vi "BaseProvider_Configuration.vi"(1 "ClassRef/ClassPath(If empty Configuration default will be modified)":variant, 3 "OnlyWireStyleConfiguration(False)":bool, 5 "Error In":errorcluster) -> (15 "SelectedWireStyleIndex":i32, 19 "Error Out":errorcluster)   [LabVIEW 2020]
uses:
  Common/LvIcon_class/GDSLvIcon_ColorControl.ctl
  SubVIs/GOOP_WirePattern.ctl
  Common/ScriptingFunctions/Scripting_ConnectorPanePatternType.ctl
  BaseProvider_SubVIs/BaseProvider_WireStyleType.ctl
  SubVIs/GOOP_WireConfigurationType.ctl
  <vilib>/Utility/miscctls.llb/LVPositionTypeDef.ctl
  <vilib>/Utility/miscctls.llb/LVBoundsTypeDef.ctl
  Common/CommonVIs/CommonVIs_ClassIconSelection_Action.ctl
  BaseProvider_SubVIs/BaseProvider_FileNamingOption.ctl
panel:
  in  "File naming option":T1(ring)
  in  "WireStyleList":T2[](array[typedef])
  in  "DiscardChanges":bool
  in  "Update/AddWireStyle":bool
  in  "DeleteWireStyle":bool
  in  "Down":bool
  in  "Up":bool
  in  "WireStyleName":string caption="Selected Wire Style Name"
  out "ProductPicture":picture
  out "IconSelection":picture
  out "Icon":picture
  in  "_Dice":cluster{"Boolean 2":bool, "Dice 2":bool}
  in  "_DefaultConnectorPanePattern":T3 caption="Default Connector Pane Pattern" items=["4x4x4", "5x6x5", "6x8x6"]
  in  "_HelpDefaultConfiguration":bool
  in  "_Help":bool
  out "_ClassItemIconApperance":string caption="Class Item Icon Appearance"
  out "_WireApperance":string
  in  "_SetToDefaultForAllClasses":bool caption="Set this to default\nfor all future classes"
  in  "_Cancel":bool
  out "_Preview":picture caption="Preview"
  in  "_Icon":u16(ring) caption="Icon" items=["BlueFull", "BlueFrame", "InterfaceBlue", "BlueCircle", "BrownFull", "BrownFrame", "InterfaceBrown", "BrownCircle", "BurgundyFull", "BurgundyFrame", "InterfaceBurgundy", "BurgundyCircle", "CyanFull", "CyanFrame", "InterfaceCyan", "CyanCircle", "DarkBlueFull", "DarkBlueFrame", "InterfaceDarkBlue", "DarkBlueCircle", "ForestGreenFull", "ForestGreenFrame", "InterfaceForestGreen", "ForestGreenCircle", "GrayFull", "GrayFrame", "InterfaceGray", "GrayCircle", "GreenFull", "GreenFrame", "InterfaceGreen", "GreenCircle", "LightGreenFull", "LightGreenFrame", "InterfaceLightGreen", "LightGreenCircle", "LightRedFull", "LightRedFrame", "InterfaceLightRed", "LightRedCircle", "PinkFull", "PinkFrame", "InterfacePink", "PinkCircle", "PurpleFull", "PurpleFrame", "InterfacePurple", "PurpleCircle", "RedFull", "RedFrame", "InterfaceRed", "RedCircle", "YellowFull", "YellowFrame", "InterfaceYellow", "YellowCircle"]
  in  "_TunnelsAndTerminalsColors":T4 caption="Tunnels and \nTerminals Colors"
  in  "_CenterColor2":T4 caption="Pattern Colors"
  in  "_CenterColor1":T4 caption="Pattern Colors"
  in  "_CenterPattern":T5 caption="Center pattern"
  in  "_EdgeColor":T4 caption="Edge color"
  in  "_CenterThickness":T6(ring) caption="Center thickness"
  in  "_EdgeThickness":T7(ring) caption="Edge thickness"
  out "Wire preview":picture
  in  "_Done":bool
  # "Wire Configuration"
  # "Wire Appearance"
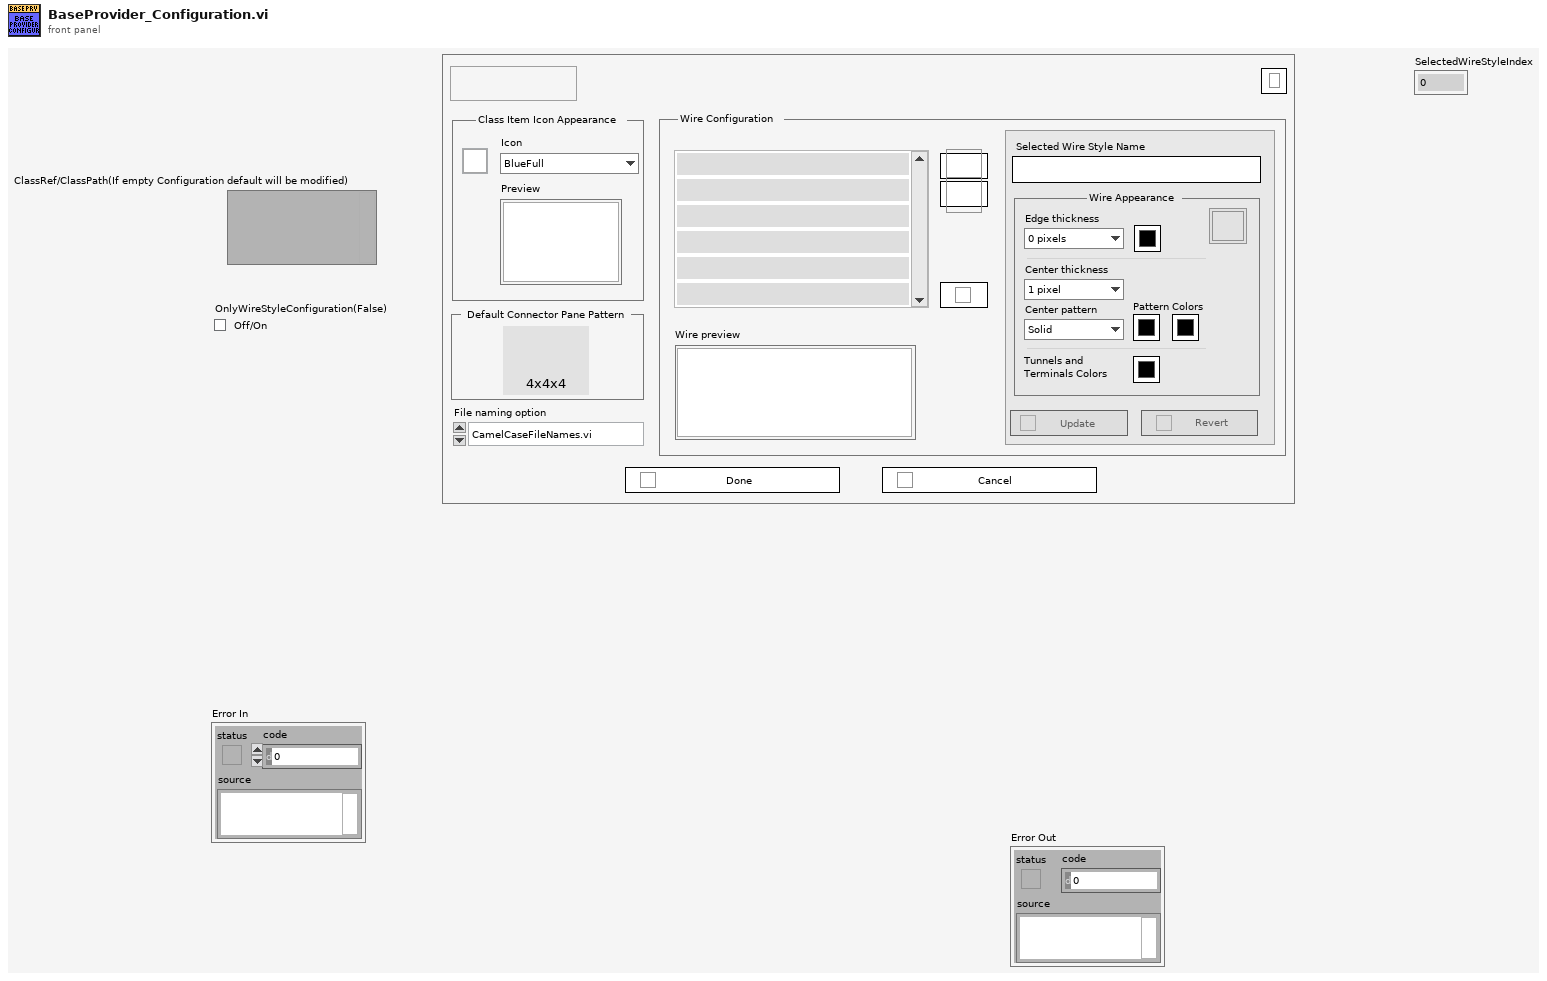
[diagram p1: front panel]
types:
  T1 = enum16{"CamelCaseFileNames.vi", "File Names With Spaces.vi", "File_Names_With_Underscores"}
  T2 = typedef "BaseProvider_WireStyleType.ctl" = cluster{"Boolean":bool, "Wire":picture, "Name":string, "Status":u16}
  T3 = typedef "Scripting_ConnectorPanePatternType.ctl" = u16
  T4 = typedef "GDSLvIcon_ColorControl.ctl" = cluster{"Decal":bool, "Color":u32}
  T5 = typedef "GOOP_WirePattern.ctl" = enum16{"Solid", "Large dash", "Small dash"}
  T6 = enum16{"1 pixel", "2 pixels", "3 pixels", "4 pixels", "5 pixels"}
  T7 = enum16{"0 pixels", "1 pixel", "2 pixels", "3 pixels"}
  T8 = typedef "GOOP_WireConfigurationType.ctl" = cluster{"Edge thickness":i32, "Edge color":u32, "Center thickness":i32, "Center pattern":T5, "CenterColor1":u32, "CenterColor2":u32, "Tunnels and terminals colors":u32}
  T9 = cluster{"FirstTime":bool, "ClassRef":refnum<vi>, "ClassRefCreated":bool, "CurrentWireStyle":T8, "DefaultIndex":i32, "SelectedWireStyleIndex":i32, "StartWireStyleIndex":i32}
  T10 = typedef "LVPositionTypeDef.ctl" = cluster{"Left":i32, "Top":i32}
  T11 = typedef "LVBoundsTypeDef.ctl" = cluster{"Width":u32, "Height":u32}
  T12 = typedef "BaseProvider_FileNamingOption.ctl" = enum16{"CamelCase", "Space", "Underscore"}
  T13 = typedef "BaseProvider_IniFileSettings.ctl" = cluster{"ClassFolderSuffix":string, "InterfaceFolderSuffix":string, "InterfaceIcon":string, "FileNamingOption":T12, "DynamicDispatchStartValue":bool, "UseGetSetForPropertyNodeMethods":bool}
  T14 = typedef "GDSLvCLass_ClassSettingsType.ctl" = cluster{"ClassProviderName":string, "ClassTemplateUsed":string, "ClassTemplateVersion":string, "ClassDescription":string, "PlugIns":T15[], "ConnectorPanePattern":string}
  T15 = typedef "GDSLvClass_PlugIn.ctl" = cluster{"Type":T16, "ID":string, "Version":string, "Path":path, "Name":string, "Data":variant}
  T16 = typedef "GDSLvClass_PlugInTypes.ctl" = enum16{"DesignPattern", "MethodTypes"}
  T17 = cluster{"Foreground Color":u32, "Background Color":u32, "Fill Pattern":cluster{"Row 0":u8, "Row 1":u8, "Row 2":u8, "Row 3":u8, "Row 4":u8, "Row 5":u8, "Row 6":u8, "Row 7":u8}, "Width":i16, "Mode":enum16{"Copy", "Or", "Exclusive Or", "Bit Clear", "Not Copy", "Not Or", "Nor Exclusive Or", "Not Bit Clear"}, "Style":enum32{"Solid", "Dash", "Dot", "Dash Dot", "Dash Dot Dot"}, "Fill Rule":enum32{"Even Odd", "Winding"}, "End Caps":enum32{"Default", "Flat"}}[]
  T18 = enum8{"Enabled", "Disabled", "Disabled and Grayed Out"}
  T19 = typedef "imagedata.ctl" = cluster{"image type":i32, "image depth":i32, "image":u8[], "mask":u8[], "colors":u32[], "Rectangle":cluster{"left":i16, "top":i16, "right":i16, "bottom":i16}}
  T20 = typedef "CommonVIs_ClassIconSelection_Action.ctl" = enum16{"All", "Non Interface", "Only Interface"}
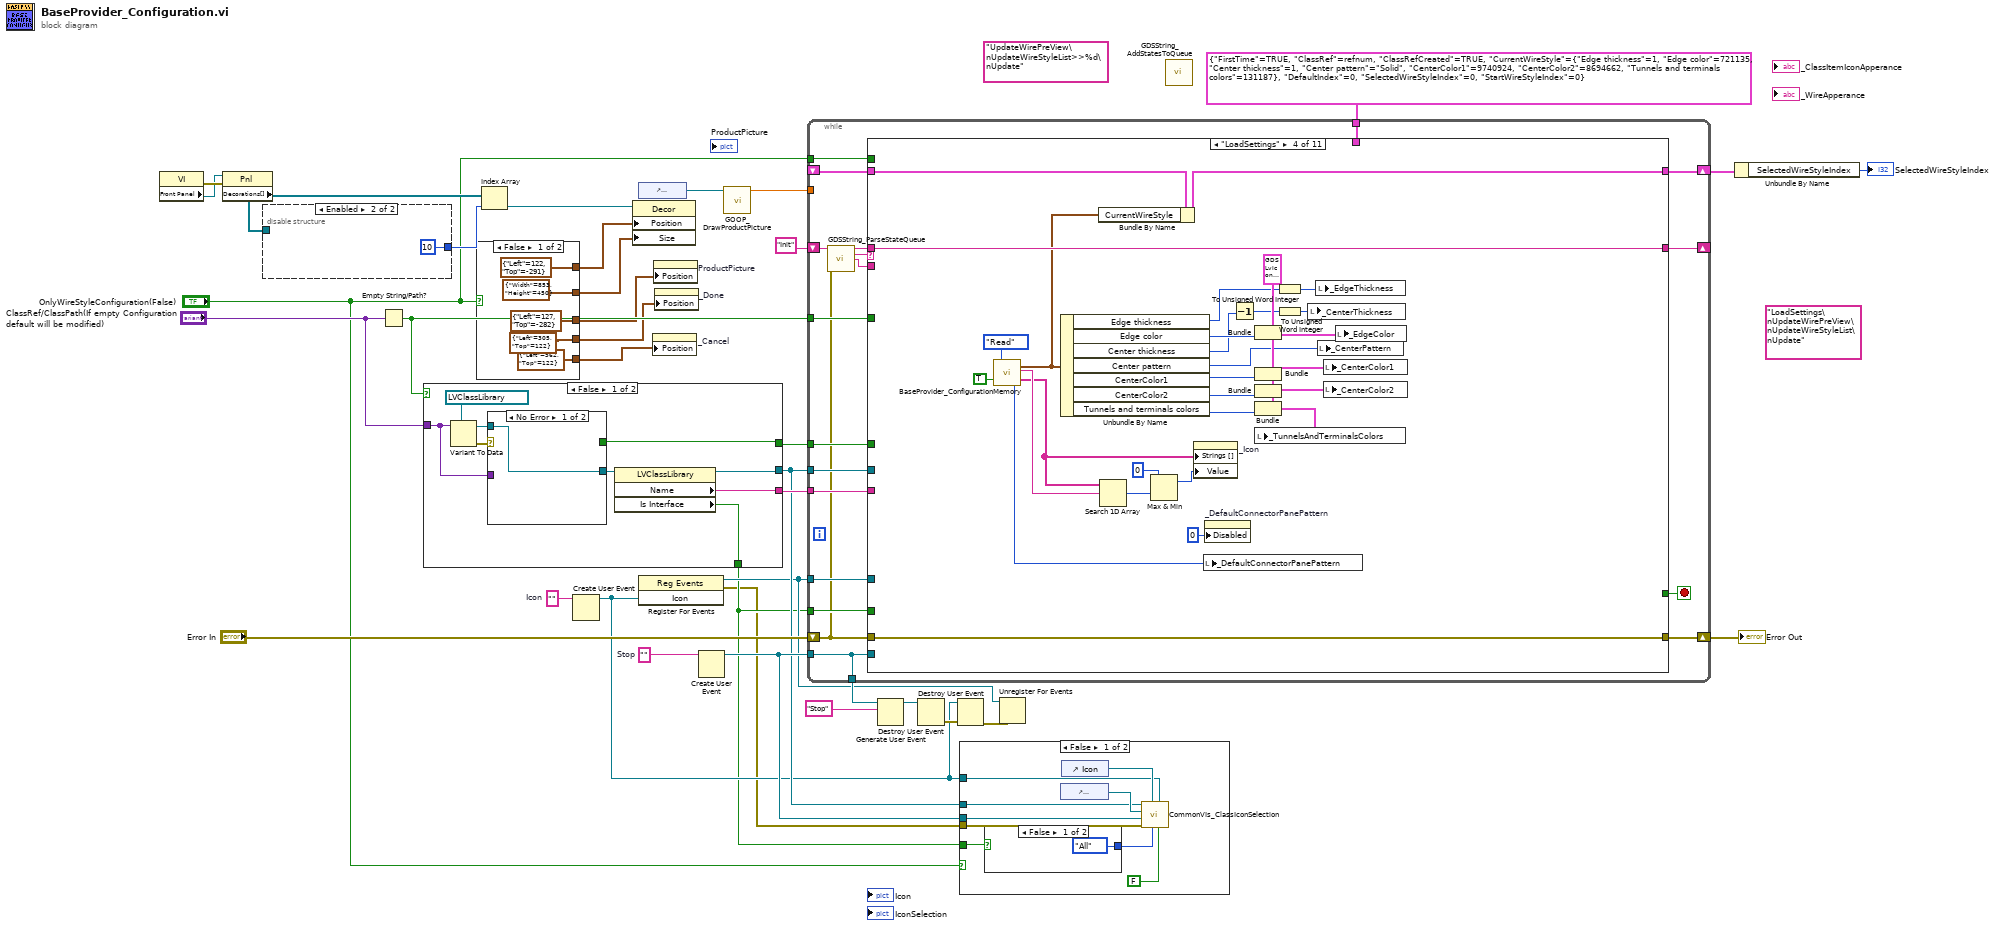
[diagram p0: block diagram]
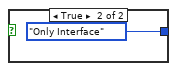
[diagram p2: hidden frame]
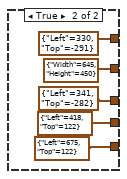
[diagram p4: hidden frame]
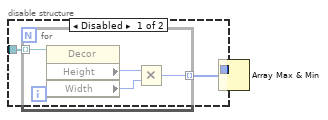
[diagram p5: hidden frame]
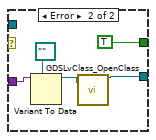
[diagram p6: hidden frame]
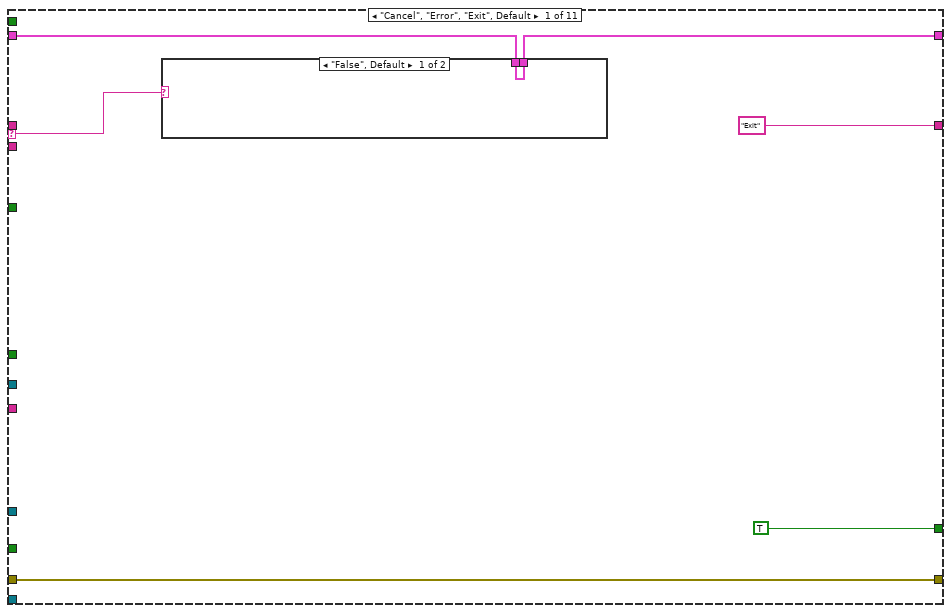
[diagram p8: hidden frame]
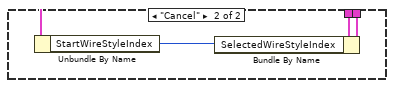
[diagram p9: hidden frame]
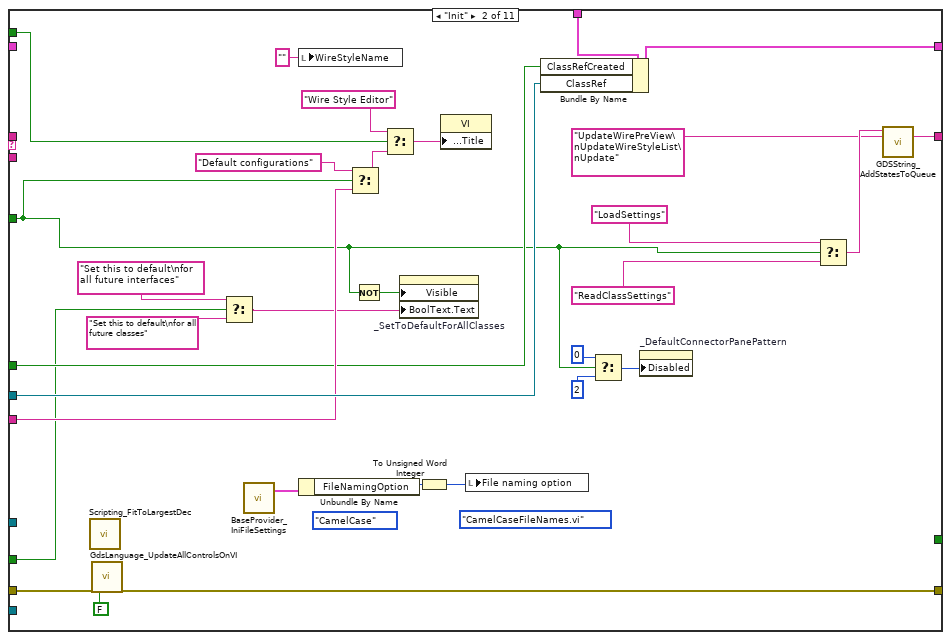
[diagram p10: hidden frame]
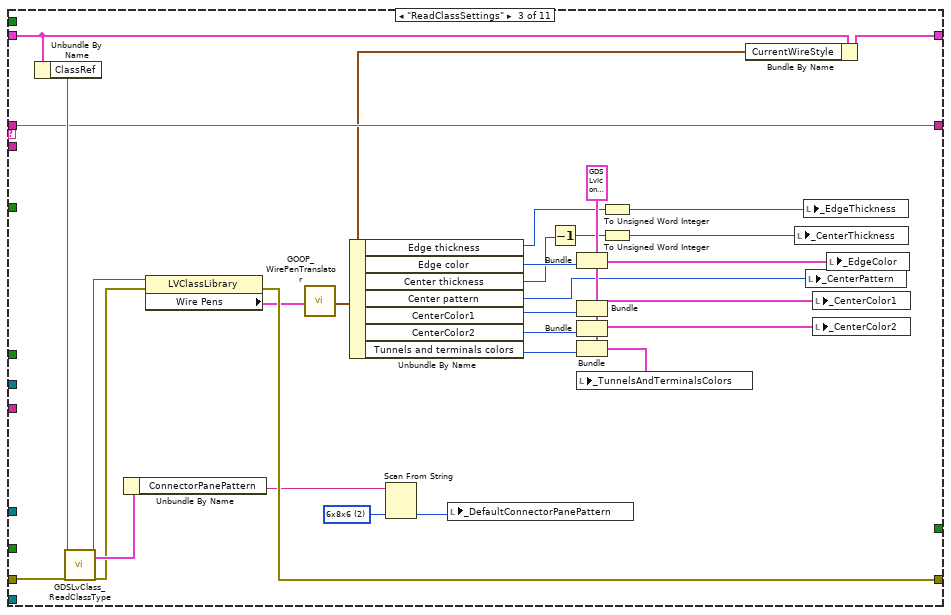
[diagram p11: hidden frame]
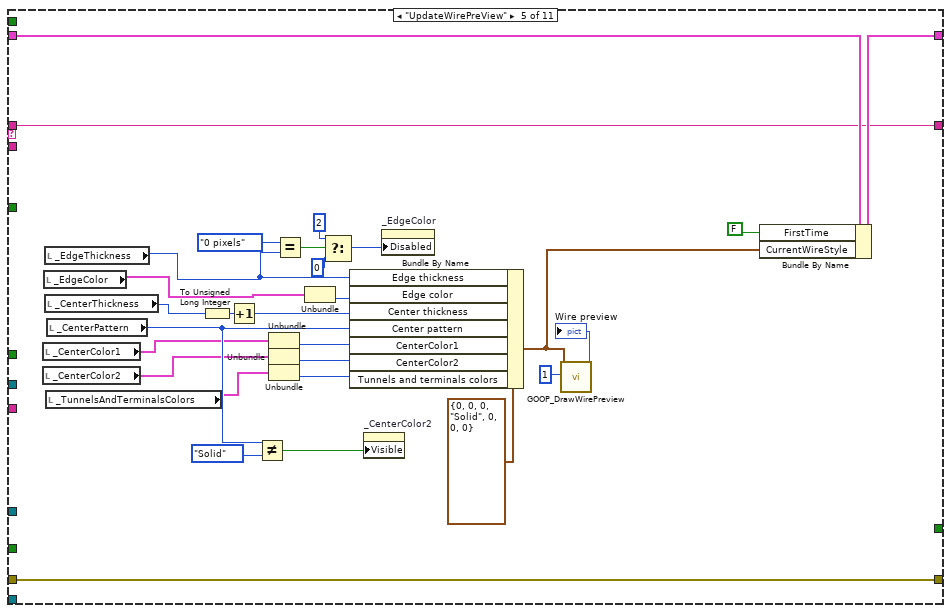
[diagram p12: hidden frame]
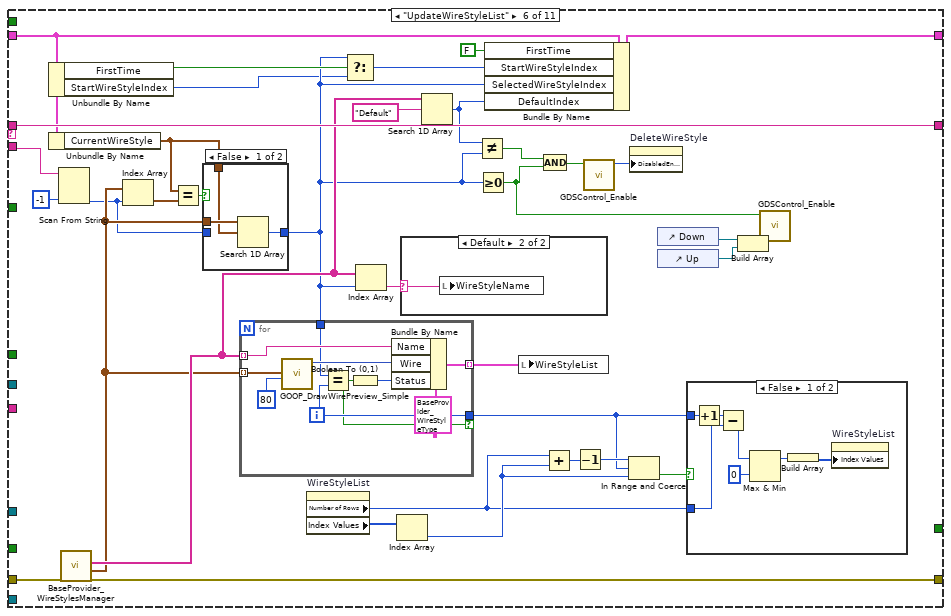
[diagram p13: hidden frame]
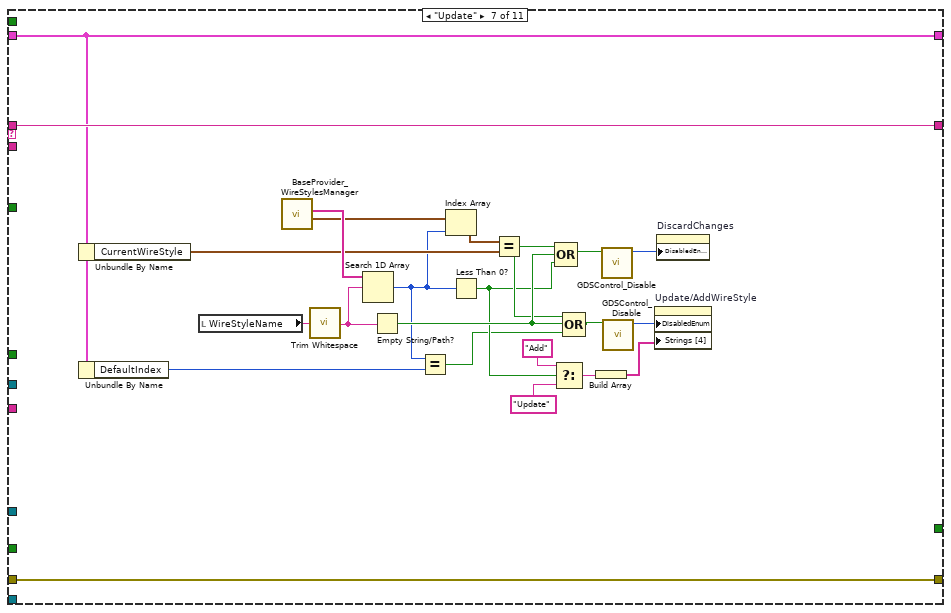
[diagram p17: hidden frame]
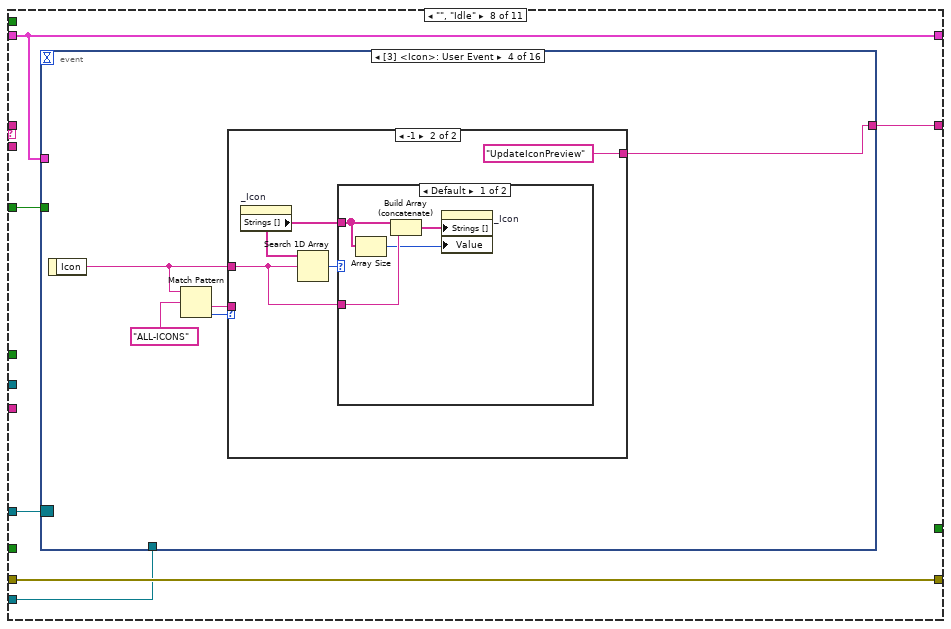
[diagram p18: hidden frame]
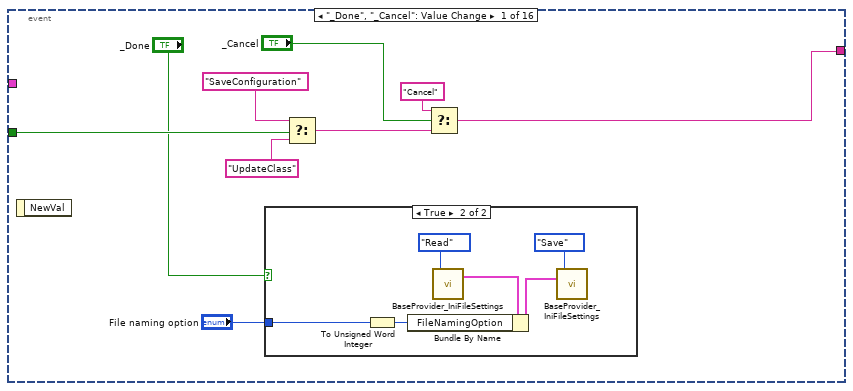
[diagram p19: hidden frame]
diagram:
  (unwired) "LoadSettings\nUpdateWirePreView\nUpdateWireStyleList\nUpdate"
  (unwired) "UpdateWirePreView\nUpdateWireStyleList>>%d\nUpdate"
  w23 = ""  # Icon
  w26 = ""  # Stop
  n1 = property on="Property Node" class="VI"() -> (error out=w13:errorcluster, "Front Panel"=w12:refnum<vi>)  [unwired: 2 in, 1 out]
  n2 = property on="Property Node" class="Pnl"(reference=w12, error in=w13) -> ("Decorations[]"=w10:refnum<vi>[])  [unwired: 2 out]
  n3 = disable-structure shown="Enabled" {
    disable-tunnel: w10 -> [w38 _]
    disable-tunnel: [_ 10 ("index")] -> w9
    frame Disabled {
      n4 = for {
        tunnel: w38 -> [w42] mode=indexing
        tunnel: [w39] -> w37 mode=indexing
        n5 = property on="Property Node" class="Decor"(reference=w42) -> ("Height"=w41:u32, "Width"=w40:u32)  [unwired: 1 in, 2 out]
        n6 = Multiply(x=w41, y=w40) -> (x*y=w39:u32)
      }
      n7 = Array Max & Min(array=w37) -> ()  [unwired: 4 out]
    }
    frame Enabled {
    }
  }
  n8 = Empty String/Path?(string/path="ClassRef/ClassPath(If empty Configuration default will be modified)") -> (empty?=w28:bool)
  n9 = case shown="False" w28 {
    tunnel: "ClassRef/ClassPath(If empty Configuration default will be modified)" -> [w50 _]
    tunnel: [w46 _] -> w24
    tunnel: [w48 _] -> w31
    tunnel: [w45 _] -> w30
    tunnel: [w44 _] -> w18
    frame False {
      n10 = Variant To Data(type=refnum<vi> refnum ("Class Refnum In"), Variant=w50) -> (data=w49:refnum<vi>, error out=w51:errorcluster)  [unwired: 1 in]
      n11 = case shown="No Error" w51 {
        tunnel: w50 -> [_ w58]
        tunnel: [w53 w55] -> w47
        tunnel: w49 -> [w53 _]
        tunnel: [_ TRUE] -> w48
        frame No Error {
        }
        frame Error {
          n12 = Variant To Data(type=path "", Variant=w58) -> (data=w56:path)  [unwired: 1 in, 1 out]
          n13 = call "GDSLvClass_OpenClass.vi"("ClassToOpen"=w56) -> ("LVClass.Open"=w55:refnum<vi>)  [unwired: 17 in, 1 out]
        }
      }
      n14 = property class="LVClassLibrary"(reference=w47) -> (reference out=w46:refnum<vi>, "Name"=w45:string, "Is Interface"=w44:bool)  [unwired: 1 in, 1 out]
    }
    frame True {
    }
  }
  n15 = case shown="False" "OnlyWireStyleConfiguration(False)" {
    tunnel: [T10 {"Left"=122, "Top"=-291} ("Position") T10 {"Left"=330, "Top"=-291} ("Position")] -> w8
    tunnel: [T11 {"Width"=853, "Height"=450} ("Size") T11 {"Width"=645, "Height"=450} ("Size")] -> w7
    tunnel: [T10 {"Left"=127, "Top"=-282} ("Position") T10 {"Left"=341, "Top"=-282} ("Position")] -> w6
    tunnel: [T10 {"Left"=305, "Top"=122} ("Position 2") T10 {"Left"=418, "Top"=122} ("Position 2")] -> w5
    tunnel: [T10 {"Left"=562, "Top"=122} ("Position 3") T10 {"Left"=675, "Top"=122} ("Position 3")] -> w4
    frame False {
    }
    frame True {
    }
  }
  n16 = Index Array(array=w10, index=w9) -> (element=w11:refnum<vi>)
  n17 = Create User Event(user event datatype=w23) -> (user event=w19:refnum<user-event>)  [unwired: 1 in, 1 out]
  n18 = property on="Property Node" class="Decor"(reference=w11, "Position"=w8, "Size"=w7) -> ()  [unwired: 1 in, 2 out]
  n19 = control-ref of="ProductPicture"() -> (w16:refnum<vi>)
  n20 = register-events(w19) -> (reference out=w22:refnum<event-registration>, error out=w17:errorcluster)  [unwired: 2 in]
  n21 = property on="_Cancel" class="Bool"("Position"=w4) -> ()  [unwired: 2 in, 2 out]
  n22 = property on="ProductPicture" class="Pict"("Position"=w6) -> ()  [unwired: 2 in, 2 out]
  n23 = property on="_Done" class="Bool"("Position"=w5) -> ()  [unwired: 2 in, 2 out]
  n24 = Create User Event(user event datatype=w26) -> (user event=w27:refnum<user-event>)  [unwired: 1 in, 1 out]
  n25 = call "GOOP_DrawProductPicture.vi"("ProductPictureControl"=w16) -> ("Zoom Factor"=w15:sgl)  [unwired: 10 in]
  n26 = while {
    shift-right: [w87] -> w34
    shift-left: "Error In" -> [w76]
    shift-right: [w72] -> _
    shift-left: "Init" -> [w77]
    shift-right: [w86] -> w3
    shift-left: _ -> [w85]
    tunnel: w27 -> [w80]
    tunnel: [w80] -> w32
    tunnel: w28 -> [w84]
    tunnel: w24 -> [w83]
    tunnel: w31 -> [w82]
    tunnel: w30 -> [w81]
    tunnel: w22 -> [w79]
    tunnel: w18 -> [w78]
    tunnel: w15 -> [_]
    tunnel: T9 {"FirstTime"=TRUE, "ClassRef"=refnum, "ClassRefCreated"=TRUE, "CurrentWireStyle"={"Edge thickness"=1, "Edge color"=721135, "Center thickness"=1, "Center pattern"=enum."Solid", "CenterColor1"=9740924, "CenterColor2"=8694662, "Tunnels and terminals colors"=131187}, "DefaultIndex"=0, "SelectedWireStyleIndex"=0, "StartWireStyleIndex"=0} -> [w70]
    tunnel: "OnlyWireStyleConfiguration(False)" -> [w69]
    stop <- w71 stop-if-true
    n27 = call "GDSString_ParseStateQueue.vi"("State Queue"=w77, "Error In (no error)"=w76) -> ("Remaining States"=w74:string, "Current State"=w75:string, "Arguments"=w73:string)  [unwired: 9 in, 2 out]
    n28 = case shown="\"LoadSettings\"" w75 {
      selector: w75 -> [w88 _ _ _ _ _ _ _ _ _ _]
      tunnel: w76 -> [w93 w123 w139 w171 w193 w251 w286 w301 w461 w515 w536]
      tunnel: [w93 w122 w156 w171 w193 w248 w286 w301 w467 w515 w536] -> w87
      tunnel: ["Exit" w107 w132 w163 w187 w250 w296 w302 w494 "Idle" "Exit"] -> w72
      tunnel: [w90 w125 w131 w161 w192 w237 w277 w297 w489 w516 w524] -> w86
      tunnel: w85 -> [w89 _ w157 w160 w188 w220 w277 w297 w489 w516 w534]
      tunnel: w84 -> [_ w113 _ _ _ _ _ w300 _ _ _]
      tunnel: w83 -> [_ w120 _ _ _ _ _ _ _ _ _]
      tunnel: w82 -> [_ w118 _ _ _ _ _ _ _ _ _]
      tunnel: w81 -> [_ w119 _ _ _ _ _ _ _ _ _]
      tunnel: w80 -> [_ _ _ _ _ _ _ w298 _ _ _]
      tunnel: w79 -> [_ _ _ _ _ _ _ w299 _ _ _]
      tunnel: w78 -> [_ w117 _ _ _ _ _ _ _ _ w531]
      tunnel: w74 -> [_ _ w132 w163 w187 w250 w296 _ _ _ _]
      tunnel: w73 -> [_ _ _ _ _ w227 _ _ _ _ _]
      tunnel: [TRUE _ _ _ _ _ _ _ _ _ _] -> w71
      tunnel: w70 -> [_ w106 _ _ _ _ _ _ _ _ _]
      tunnel: w69 -> [_ w101 _ _ _ _ _ _ _ _ _]
      frame "Cancel", "Error", "Exit", Default {
        n29 = case shown="\"False\", Default" w88 {
          tunnel: [w94 w97] -> w90
          tunnel: w89 -> [w94 w96]
          frame "False", Default {
          }
          frame "Cancel" {
            n30 = Unbundle By Name(w96) -> ("StartWireStyleIndex"=w95:i32)
            n31 = Bundle By Name(cluster=w96, "SelectedWireStyleIndex"=w95) -> (w97:T9)
          }
        }
      }
      frame "Init" {
        (unwired) T1."CamelCaseFileNames.vi" ("File naming option")
        (unwired) BaseProvider_FileNamingOption."CamelCase" ("FileNamingOption")
        n32 = call "Scripting_FitToLargestDec.vi"() -> ()  [unwired: 6 in, 2 out]
        n33 = call "GdsLanguage_UpdateAllControlsOnVI.vi"("error in (no error)"=w123, "CreateLanguageFile(Use this to create a languageFile)"=FALSE) -> ("error out"=w122:errorcluster)  [unwired: 16 in, 1 out]
        n34 = Select(t="Set this to default\nfor all future interfaces", s=w117, f="Set this to default\nfor all future classes") -> (s? t:f=w114:string)
        n35 = call "BaseProvider_IniFileSettings.vi"() -> ("IniFileSettings"=w100:T13)  [unwired: 18 in, 1 out]
        n36 = local write "WireStyleName"("" ("WireStyleName")) -> ()
        n37 = Unbundle By Name(w100) -> ("FileNamingOption"=w99:T12)
        n38 = Select(t="Default configurations", s=w113, f=w119) -> (s? t:f=w104:string)
        n39 = Not(x=w113) -> (.not. x?=w124:bool)
        n40 = Select(t="Wire Style Editor", s=w101, f=w104) -> (s? t:f=w103:string)
        n41 = property on="_SetToDefaultForAllClasses" class="Bool (strict)"("Visible"=w124, "BoolText.Text"=w114) -> ()  [unwired: 2 in, 2 out]
        n42 = To Unsigned Word Integer(number=w99) -> (unsigned 16bit integer=w98:u16)
        n43 = property class="VI"("Front Panel.Title"=w103) -> ()  [unwired: 2 in, 2 out]
        n44 = local write "File naming option"(w98) -> ()
        n45 = Bundle By Name(cluster=w106, "ClassRefCreated"=w118, "ClassRef"=w120) -> (w125:T9)
        n46 = Select(t=u8 0 ("Disabled"), s=w113, f=u8 2 ("Disabled")) -> (s? t:f=w111:u8)
        n47 = property on="_DefaultConnectorPanePattern" class="Ring (strict)"("Disabled"=w111) -> ()  [unwired: 2 in, 2 out]
        n48 = Select(t="LoadSettings", s=w113, f="ReadClassSettings") -> (s? t:f=w109:string)
        n49 = call "GDSString_AddStatesToQueue.vi"("State(s) in Front (\"\")"=w109, "State(s) in (\"\")"="UpdateWirePreView\nUpdateWireStyleList\nUpdate") -> ("States Out"=w107:string)  [unwired: 13 in]
      }
      frame "ReadClassSettings" {
        w136 = T3 2 items=["4x4x4", "5x6x5", "6x8x6"] ("Pattern")
        w149 = T4 {"Decal"=FALSE, "Color"=11184810} ("Edge color")
        n50 = Unbundle By Name(w157) -> ("ClassRef"=w138:refnum<vi>)
        n51 = call "GDSLvClass_ReadClassType.vi"("Class Refnum In"=w138, "error in (no error)"=w139) -> ("Class Refnum Out"=w133:refnum<vi>, "ClassSettings"=w137:T14, "error out"=w129:errorcluster)  [unwired: 15 in]
        n52 = Unbundle By Name(w137) -> ("ConnectorPanePattern"=w135:string)
        n53 = property class="LVClassLibrary"(reference=w133, error in=w129) -> (error out=w156:errorcluster, "Wire Pens"=w155:T17)  [unwired: 1 out]
        n54 = call "GOOP_WirePenTranslator.vi"("WirePensIn"=w155) -> ("WireConfigurationOut"=w130:T8)  [unwired: 17 in, 1 out]
        n55 = Unbundle By Name(w130) -> ("Edge thickness"=w141:i32, "Edge color"=w154:u32, "Center thickness"=w144:i32, "Center pattern"=w145:T5, "CenterColor1"=w153:u32, "CenterColor2"=w152:u32, "Tunnels and terminals colors"=w151:u32)
        n56 = Scan From String(input string=w135, default 1=w136) -> (output 1=w134:T3)  [unwired: 3 in, 3 out]
        n57 = local write "_DefaultConnectorPanePattern"(w134) -> ()
        n58 = Decrement(x=w144) -> (x-1=w143:i32)
        n59 = Bundle(cluster=w149, "Color"=w154) -> (w146:T4)  [unwired: 1 in]
        n60 = Bundle(cluster=w149, "Color"=w153) -> (w147:T4)  [unwired: 1 in]
        n61 = Bundle(cluster=w149, "Color"=w152) -> (w148:T4)  [unwired: 1 in]
        n62 = Bundle(cluster=w149, "Color"=w151) -> (w150:T4)  [unwired: 1 in]
        n63 = local write "_TunnelsAndTerminalsColors"(w150) -> ()
        n64 = To Unsigned Word Integer(number=w141) -> (unsigned 16bit integer=w140:u16)
        n65 = To Unsigned Word Integer(number=w143) -> (unsigned 16bit integer=w142:u16)
        n66 = Bundle By Name(cluster=w157, "CurrentWireStyle"=w130) -> (w131:T9)
        n67 = local write "_CenterThickness"(w142) -> ()
        n68 = local write "_EdgeThickness"(w140) -> ()
        n69 = local write "_CenterPattern"(w145) -> ()
        n70 = local write "_CenterColor1"(w147) -> ()
        n71 = local write "_CenterColor2"(w148) -> ()
        n72 = local write "_EdgeColor"(w146) -> ()
      }
      frame "LoadSettings" {
        w181 = T4 {"Decal"=FALSE, "Color"=11184810} ("Edge color")
        n73 = call "BaseProvider_ConfigurationMemory.vi"("Filter_Icons"=TRUE, "Action"=enum16{"Read", "Load", "Save"}."Read") -> ("PatternOut"=w166:T3, "WireConfigurationOut"=w162:T8, "IconOut"=w169:string, "ClassItemIconNames"=w159:string[])  [unwired: 11 in, 3 out]
        n74 = Unbundle By Name(w162) -> ("Edge thickness"=w173:i32, "Edge color"=w186:u32, "Center thickness"=w176:i32, "Center pattern"=w177:T5, "CenterColor1"=w185:u32, "CenterColor2"=w184:u32, "Tunnels and terminals colors"=w183:u32)
        n75 = Bundle By Name(cluster=w160, "CurrentWireStyle"=w162) -> (w161:T9)
        n76 = Search 1D Array(1D array=w159, element=w169) -> (index of element=w167:i32)  [unwired: 1 in]
        n77 = Max & Min(x=0, y=w167) -> (max(x,y)=w158:i32)  [unwired: 1 out]
        n78 = property on="_Icon" class="Ring (strict)"("Strings []"=w159, "Value"=w158) -> ()  [unwired: 2 in, 2 out]
        n79 = local write "_DefaultConnectorPanePattern"(w166) -> ()
        n80 = property on="_DefaultConnectorPanePattern" class="Ring (strict)"("Disabled"=u8 0) -> ()  [unwired: 2 in, 2 out]
        n81 = Decrement(x=w176) -> (x-1=w175:i32)
        n82 = Bundle(cluster=w181, "Color"=w186) -> (w178:T4)  [unwired: 1 in]
        n83 = Bundle(cluster=w181, "Color"=w185) -> (w179:T4)  [unwired: 1 in]
        n84 = Bundle(cluster=w181, "Color"=w184) -> (w180:T4)  [unwired: 1 in]
        n85 = Bundle(cluster=w181, "Color"=w183) -> (w182:T4)  [unwired: 1 in]
        n86 = local write "_TunnelsAndTerminalsColors"(w182) -> ()
        n87 = To Unsigned Word Integer(number=w173) -> (unsigned 16bit integer=w172:u16)
        n88 = To Unsigned Word Integer(number=w175) -> (unsigned 16bit integer=w174:u16)
        n89 = local write "_CenterThickness"(w174) -> ()
        n90 = local write "_EdgeThickness"(w172) -> ()
        n91 = local write "_CenterPattern"(w177) -> ()
        n92 = local write "_CenterColor1"(w179) -> ()
        n93 = local write "_CenterColor2"(w180) -> ()
        n94 = local write "_EdgeColor"(w178) -> ()
      }
      frame "UpdateWirePreView" {
        n95 = local read "_CenterColor1"() -> (w196:T4)
        n96 = local read "_CenterColor2"() -> (w195:T4)
        n97 = local read "_EdgeColor"() -> (w199:T4)
        n98 = local read "_EdgeThickness"() -> (w200:T7)
        n99 = local read "_CenterThickness"() -> (w198:T6)
        n100 = local read "_TunnelsAndTerminalsColors"() -> (w194:T4)
        n101 = local read "_CenterPattern"() -> (w197:T5)
        n102 = To Unsigned Long Integer(number=w198) -> (unsigned 32bit integer=w215:u32)
        n103 = Increment(x=w215) -> (x+1=w208:u32)
        n104 = Not Equal?(x=w197, y=GOOP_WirePattern."Solid") -> (x != y?=w190:bool)
        n105 = Unbundle(w196) -> ("Color"=w206:u32)  [unwired: 1 out]
        n106 = Unbundle(w195) -> ("Color"=w207:u32)  [unwired: 1 out]
        n107 = Unbundle(w194) -> ("Color"=w204:u32)  [unwired: 1 out]
        n108 = Equal?(x=T7."0 pixels", y=w200) -> (x = y?=w210:bool)
        n109 = Unbundle(w199) -> ("Color"=w205:u32)  [unwired: 1 out]
        n110 = Select(t=u8 2 ("Disabled"), s=w210, f=u8 0) -> (s? t:f=w212:u8)
        n111 = Bundle By Name(cluster=T8 {"Edge thickness"=0, "Edge color"=0, "Center thickness"=0, "Center pattern"=enum."Solid", "CenterColor1"=0, "CenterColor2"=0, "Tunnels and terminals colors"=0} ("WireConfiguration"), "Edge thickness"=w200, "Edge color"=w205, "Center thickness"=w208, "Center pattern"=w197, "CenterColor1"=w206, "CenterColor2"=w207, "Tunnels and terminals colors"=w204) -> (w189:T8)
        n112 = property on="_CenterColor2" class="Clust (strict)"("Visible"=w190) -> ()  [unwired: 2 in, 2 out]
        n113 = property on="_EdgeColor" class="Clust (strict)"("Disabled"=w212) -> ()  [unwired: 2 in, 2 out]
        n114 = call "GOOP_DrawWirePreview.vi"("WireConfiguration"=w189, "Zoom"=1) -> ("Picture"=→"Wire preview":picture)  [unwired: 16 in, 1 out]
        n115 = Bundle By Name(cluster=w188, "FirstTime"=FALSE, "CurrentWireStyle"=w189) -> (w192:T9)
      }
      frame "UpdateWireStyleList" {
        n116 = Unbundle By Name(w220) -> ("FirstTime"=w219:bool, "StartWireStyleIndex"=w216:i32)
        n117 = Unbundle By Name(w220) -> ("CurrentWireStyle"=w225:T8)
        n118 = Scan From String(input string=w227, default 1=-1 ("default value 1")) -> (output 1=w222:i32)  [unwired: 3 in, 3 out]
        n119 = call "BaseProvider_WireStylesManager.vi"("error in (no error)"=w251) -> ("error out"=w248:errorcluster, "AllWireConfigurations"=w228:T8[], "AllWireConfigurations(Names)"=w239:string[])  [unwired: 7 in, 1 out]
        n120 = Index Array(array=w228, index=w222) -> (element=w224:T8)
        n121 = Equal?(x=w225, y=w224) -> (x = y?=w223:bool)
        n122 = case shown="False" w223 {
          tunnel: [w254 w255] -> w218
          tunnel: w228 -> [w253 _]
          tunnel: w225 -> [w252 _]
          tunnel: w222 -> [_ w255]
          frame False {
            n123 = Search 1D Array(1D array=w253, element=w252) -> (index of element=w254:i32)  [unwired: 1 in]
          }
          frame True {
          }
        }
        n124 = for {
          tunnel: w239 -> [w269] mode=indexing
          tunnel: w228 -> [w272] mode=indexing
          tunnel: [w268] -> w249 mode=indexing
          tunnel: w218 -> [w267]
          tunnel: [w265] -> w241 if=w264
          i -> [w265]
          n125 = call "GOOP_DrawWirePreview_Simple.vi"("WireLength(100px)"=i16 80, "WireConfiguration"=w272) -> ("WirePictureOut"=w270:picture)  [unwired: 5 in, 4 out]
          n126 = Equal?(x=w267, y=w265) -> (x = y?=w264:bool)
          n127 = Boolean To (0,1)(Boolean=w264) -> (0, 1=w266:i16)
          n128 = Bundle By Name(cluster=T2 {"Boolean"=FALSE, "Wire"=bytes[0], "Name"="", "Status"=0} ("Cluster 2"), "Name"=w269, "Wire"=w270, "Status"=w266) -> (w268:T2)
        }
        n129 = property on="WireStyleList" class="Arr (strict)"() -> ("Number of Rows"=w240:u32, "Index Values"=w246:u32[])  [unwired: 2 in, 2 out]
        n130 = Select(t=w218, s=w219, f=w216) -> (s? t:f=w217:i32)
        n131 = Index Array(array=w239, index=w218) -> (element=w247:string)
        n132 = Index Array(array=w246) -> (element=w245:u32)  [unwired: 1 in]
        n133 = case shown="Default" w247 {
          selector: w247 -> [_ w263]
          frame "" {
          }
          frame Default {
            n134 = local write "WireStyleName"(w263) -> ()
          }
        }
        n135 = Search 1D Array(1D array=w239, element="Default") -> (index of element=w236:i32)  [unwired: 1 in]
        n136 = Not Equal?(x=w236, y=w218) -> (x != y?=w235:bool)
        n137 = Greater Or Equal To 0?(x=w218) -> (x >= 0?=w232:bool)
        n138 = Bundle By Name(cluster=w220, "FirstTime"=FALSE, "StartWireStyleIndex"=w217, "SelectedWireStyleIndex"=w218, "DefaultIndex"=w236) -> (w237:T9)
        n139 = local write "WireStyleList"(w249) -> ()
        n140 = Compound Arithmetic op=AND(w235, w232) -> (w234:bool)
        n141 = Add(x=w240, y=w245) -> (x+y=w244:u32)
        n142 = Decrement(x=w244) -> (x-1=w243:u32)
        n143 = call "GDSControl_Enable.vi"("Enable(True)"=w234) -> ("Enable Property"=w233:T18)  [unwired: 10 in]
        n144 = In Range and Coerce(upper limit=w243, x=w241, lower limit=w245) -> (In Range?=w242:bool)  [unwired: 1 out]
        n145 = property on="DeleteWireStyle" class="Bool"("DisabledEnum"=w233) -> ()  [unwired: 2 in, 2 out]
        n146 = control-ref of="Down"() -> (w231:refnum<vi>)
        n147 = control-ref of="Up"() -> (w230:refnum<vi>)
        n148 = case shown="False" w242 {
          tunnel: w241 -> [w261 _]
          tunnel: w240 -> [w260 _]
          frame False {
            n149 = Increment(x=w261) -> (x+1=w256:i32)
            n150 = Subtract(x=w256, y=w260) -> (x-y=w259:u32)
            n151 = Max & Min(x=w259, y=u32 0) -> (max(x,y)=w257:u32)  [unwired: 1 out]
            n152 = Build Array(w257) -> (w262:u32[])
            n153 = property on="WireStyleList" class="Arr (strict)"("Index Values"=w262) -> ()  [unwired: 2 in, 2 out]
          }
          frame True {
          }
        }
        n154 = Build Array(w231, w230) -> (w229:refnum<vi>[])
        n155 = call "GDSControl_Enable.vi"("ManyControls"=w229, "Enable(True)"=w232) -> ()  [unwired: 9 in, 1 out]
      }
      frame "Update" {
        n156 = Unbundle By Name(w277) -> ("CurrentWireStyle"=w290:T8)
        n157 = Unbundle By Name(w277) -> ("DefaultIndex"=w275:i32)
        n158 = local read "WireStyleName"() -> (w295:string)
        n159 = call "BaseProvider_WireStylesManager.vi"() -> ("AllWireConfigurations"=w291:T8[], "AllWireConfigurations(Names)"=w293:string[])  [unwired: 8 in, 2 out]
        n160 = call <vilib>:"Trim Whitespace.vi"("string"=w295) -> ("trimmed string"=w292:string)  [unwired: 1 in]
        n161 = Search 1D Array(1D array=w293, element=w292) -> (index of element=w276:i32)  [unwired: 1 in]
        n162 = Empty String/Path?(string/path=w292) -> (empty?=w285:bool)
        n163 = Equal?(x=w276, y=w275) -> (x = y?=w274:bool)
        n164 = Index Array(array=w291, index=w276) -> (element=w289:T8)
        n165 = Less Than 0?(x=w276) -> (x < 0?=w282:bool)
        n166 = Equal?(x=w289, y=w290) -> (x = y?=w283:bool)
        n167 = Select(t="Add", s=w282, f="Update") -> (s? t:f=w279:string)
        n168 = Compound Arithmetic op=OR(w283, w285, w282) -> (w288:bool)
        n169 = Compound Arithmetic op=OR(w283, w285, w274) -> (w284:bool)
        n170 = Build Array(w279) -> (w278:string[])
        n171 = call "GDSControl_Disable.vi"("Disasble(True)"=w288) -> ("Enable Property"=w287:T18)  [unwired: 10 in]
        n172 = call "GDSControl_Disable.vi"("Disasble(True)"=w284) -> ("Enable Property"=w294:T18)  [unwired: 10 in]
        n173 = property on="Update/AddWireStyle" class="Bool"("DisabledEnum"=w294, "Strings [4]"=w278) -> ()  [unwired: 2 in, 2 out]
        n174 = property on="DiscardChanges" class="Bool"("DisabledEnum"=w287) -> ()  [unwired: 2 in, 2 out]
      }
      frame "", "Idle" {
        n175 = event shown="[3] <Icon>: User Event" {
          selector: w299 -> [_ _ _ _ _ _ _ _ _ _ _ _ _ _ _ _]
          dyn-events: _ -> [_ _ _ _ _ _ _ _ _ _ _ _ _ _ _ _]
          timeout: _ -> [_ _ _ _ _ _ _ _ _ _ _ _ _ _ _ _]
          tunnel: [w307 "Exit" "UpdateIconPreview" w325 "UpdateWirePreView\nUpdate" "Idle" "UpdateWirePreView\nUpdate" w356 "Update" w387 "UpdateWirePreView\nUpdateWireStyleList\nUpdate" "UpdateWirePreView\nUpdateWireStyleList\nUpdate" w432 "Idle" "Idle" "Idle"] -> w302
          tunnel: w300 -> [w305 _ _ _ _ _ _ _ _ _ _ _ _ _ _ _]
          tunnel: w298 -> [_ _ w322 _ _ _ _ _ _ _ _ _ _ _ _ _]
          tunnel: w297 -> [_ _ _ _ _ _ _ _ _ _ _ w427 w441 _ _ _]
          event "_Done", "_Cancel": Value Change {
            n176 = event-data() -> ()  [unwired: 1 in, 1 out]
            n177 = case shown="True" "_Done" {
              tunnel: "File naming option" -> [_ w312]
              frame False {
              }
              frame True {
                n178 = To Unsigned Word Integer(number=w312) -> (unsigned 16bit integer=w313:u16)
                n179 = call "BaseProvider_IniFileSettings.vi"("Action"=enum16{"Read", "Load", "Save"}."Read") -> ("IniFileSettings"=w317:T13)  [unwired: 17 in, 1 out]
                n180 = Bundle By Name(cluster=w317, "FileNamingOption"=w313) -> (w314:T13)
                n181 = call "BaseProvider_IniFileSettings.vi"("IniFileSettings"=w314, "Action"=enum16{"Read", "Load", "Save"}."Save") -> ()  [unwired: 16 in, 2 out]
              }
            }
            n182 = Select(t="SaveConfiguration", s=w305, f="UpdateClass") -> (s? t:f=w308:string)
            n183 = Select(t="Cancel", s="_Cancel", f=w308) -> (s? t:f=w307:string)
          }
          event Panel Close? {
            n184 = event-data() -> ()  [unwired: 1 in, 4 out]
            n185 = event-data("Discard?"=TRUE) -> ()  [unwired: 1 in, 1 out]
          }
          event "_Icon": Value Change {
            n186 = event-data() -> ()  [unwired: 1 in, 1 out]
            n187 = property on="_Icon" class="Ring (strict)"() -> ("Strings []"=w323:string[])  [unwired: 2 in, 2 out]
            n188 = Index Array(array=w323, index="_Icon") -> (element=w321:string)
            n189 = Generate User Event(user event=w322, event data cluster=w321) -> ()  [unwired: 2 in, 2 out]
          }
          event User Event {
            n190 = event-data() -> ("Icon"=w329:string)  [unwired: 1 in]
            n191 = Match Pattern(string=w329, regular expression="ALL-ICONS" ("string")) -> (after substring=w326:string, offset past match=w327:i32)  [unwired: 1 in, 2 out]
            n192 = case shown="-1" w327 {
              tunnel: w329 -> [_ w335]
              tunnel: w326 -> [w331 _]
              tunnel: ["Idle" "UpdateIconPreview"] -> w325
              frame 0, Default {
                n193 = Spreadsheet String To Array(format string="%s", spreadsheet string=w331, array type (2D Dbl)=string[] []) -> (array=w334:string[])  [unwired: 1 in]
                n194 = property on="_Icon" class="Ring (strict)"("Strings []"=w334) -> ()  [unwired: 2 in, 2 out]
              }
              frame -1 {
                n195 = property on="_Icon" class="Ring (strict)"() -> ("Strings []"=w336:string[])  [unwired: 2 in, 2 out]
                n196 = Search 1D Array(1D array=w336, element=w335) -> (index of element=w338:i32)  [unwired: 1 in]
                n197 = case shown="Default" w338 {
                  selector: w338 -> [_ w343]
                  tunnel: w336 -> [w340 _]
                  tunnel: w335 -> [w341 _]
                  frame Default {
                    n198 = Array Size(array=w340) -> (size(s)=w339:i32)
                    n199 = Build Array (concatenate)(w340, w341) -> (w342:string[])
                    n200 = property on="_Icon" class="Ring (strict)"("Strings []"=w342, "Value"=w339) -> ()  [unwired: 2 in, 2 out]
                  }
                  frame 0.. {
                    n201 = local write "_Icon"(w343) -> ()
                  }
                }
              }
            }
          }
          event "_EdgeThickness", "_CenterThickness": Value Change {
            n202 = event-data() -> ()  [unwired: 1 in, 1 out]
          }
          event "_Help": Value Change {
            n203 = event-data() -> ()  [unwired: 1 in, 1 out]
            n204 = call "GOOP_HelpMain.vi"() -> ()  [unwired: 12 in]
          }
          event "_Dice": Value Change {
            n205 = event-data() -> ()  [unwired: 1 in, 1 out]
            n206 = control-ref of="_TunnelsAndTerminalsColors"() -> (w353:refnum<vi>)
            n207 = control-ref of="_EdgeColor"() -> (w351:refnum<vi>)
            n208 = control-ref of="_CenterColor1"() -> (w348:refnum<vi>)
            n209 = control-ref of="_CenterColor2"() -> (w347:refnum<vi>)
            n210 = control-ref of="_CenterPattern"() -> (w352:refnum<vi>)
            n211 = control-ref of="_CenterThickness"() -> (w350:refnum<vi>)
            n212 = control-ref of="_EdgeThickness"() -> (w349:refnum<vi>)
            n213 = call "BaseProvider_RandomWireConfig.vi"("EdgeColor"=w351, "_CenterThickness"=w350, "_EdgeThickness"=w349, "_CenterColor2"=w348, "_CenterColor1"=w347, "_CenterPattern"=w352, "_TunnelsAndTerminalsColors"=w353) -> ()  [unwired: 13 in]
            n214 = local write "_Dice"(cluster{"Boolean 2":bool, "Dice":bool} {"Boolean 2"=TRUE, "Dice"=FALSE} ("Dice")) -> ()
          }
          event "WireStyleList": Value Change {
            n215 = event-data() -> ("OldVal"=w355:T2[], "NewVal"=w360:T2[])  [unwired: 1 in, 1 out]
            n216 = for {
              tunnel: w360 -> [w385] mode=indexing
              tunnel: [w384] -> w359 mode=indexing
              n217 = Unbundle By Name(w385) -> ("Boolean"=w384:bool)
            }
            n218 = Search 1D Array(1D array=w359, element=TRUE) -> (index of element=w357:i32)  [unwired: 1 in]
            n219 = case shown="0, Default" w357 {
              selector: w357 -> [w363 _]
              tunnel: [w361 _] -> w356
              tunnel: w355 -> [w366 _]
              frame 0, Default {
                w368 = T4 {"Decal"=FALSE, "Color"=11184810} ("Edge color")
                n220 = call "BaseProvider_WireStylesManager.vi"() -> ("AllWireConfigurations"=w383:T8[], "AllWireConfigurations(Names)"=w365:string[])  [unwired: 8 in, 2 out]
                n221 = local write "WireStyleList"(w366) -> ()
                n222 = Index Array(array=w365, index=w363) -> (element=w364:string)
                n223 = Index Array(array=w383, index=w363) -> (element=w367:T8)
                n224 = local write "WireStyleName"(w364) -> ()
                n225 = Unbundle By Name(w367) -> ("Edge thickness"=w370:i32, "Edge color"=w382:u32, "Center thickness"=w373:i32, "Center pattern"=w374:T5, "CenterColor1"=w381:u32, "CenterColor2"=w380:u32, "Tunnels and terminals colors"=w379:u32)
                n226 = Format Into String(format string="UpdateWirePreView\nUpdateWireStyleList>>%d\nUpdate", w363) -> (resulting string=w361:string)  [unwired: 2 in, 1 out]
                n227 = Decrement(x=w373) -> (x-1=w372:i32)
                n228 = Bundle(cluster=w368, "Color"=w382) -> (w375:T4)  [unwired: 1 in]
                n229 = Bundle(cluster=w368, "Color"=w381) -> (w376:T4)  [unwired: 1 in]
                n230 = Bundle(cluster=w368, "Color"=w380) -> (w377:T4)  [unwired: 1 in]
                n231 = Bundle(cluster=w368, "Color"=w379) -> (w378:T4)  [unwired: 1 in]
                n232 = local write "_TunnelsAndTerminalsColors"(w378) -> ()
                n233 = To Unsigned Word Integer(number=w370) -> (unsigned 16bit integer=w369:u16)
                n234 = To Unsigned Word Integer(number=w372) -> (unsigned 16bit integer=w371:u16)
                n235 = local write "_CenterThickness"(w371) -> ()
                n236 = local write "_EdgeThickness"(w369) -> ()
                n237 = local write "_CenterPattern"(w374) -> ()
                n238 = local write "_CenterColor1"(w376) -> ()
                n239 = local write "_CenterColor2"(w377) -> ()
                n240 = local write "_EdgeColor"(w375) -> ()
              }
              frame -1 {
              }
            }
          }
          event "WireStyleName": Value Change {
            n241 = event-data() -> ()  [unwired: 1 in, 6 out]
          }
          event "DiscardChanges": Value Change {
            n242 = event-data() -> ()  [unwired: 1 in, 1 out]
            n243 = local read "WireStyleName"() -> (w392:string)
            n244 = call "BaseProvider_WireStylesManager.vi"() -> ("AllWireConfigurations"=w389:T8[], "AllWireConfigurations(Names)"=w391:string[])  [unwired: 8 in, 2 out]
            n245 = call <vilib>:"Trim Whitespace.vi"("string"=w392) -> ("trimmed string"=w390:string)  [unwired: 1 in]
            n246 = Search 1D Array(1D array=w391, element=w390) -> (index of element=w388:i32)  [unwired: 1 in]
            n247 = case shown="0, Default" w388 {
              selector: w388 -> [w410 _]
              tunnel: w389 -> [w411 _]
              tunnel: ["UpdateWirePreView\nUpdate" _] -> w387
              frame 0, Default {
                w395 = T4 {"Decal"=FALSE, "Color"=11184810} ("Edge color")
                n248 = Index Array(array=w411, index=w410) -> (element=w394:T8)
                n249 = Unbundle By Name(w394) -> ("Edge thickness"=w397:i32, "Edge color"=w409:u32, "Center thickness"=w400:i32, "Center pattern"=w401:T5, "CenterColor1"=w408:u32, "CenterColor2"=w407:u32, "Tunnels and terminals colors"=w406:u32)
                n250 = Decrement(x=w400) -> (x-1=w399:i32)
                n251 = Bundle(cluster=w395, "Color"=w409) -> (w402:T4)  [unwired: 1 in]
                n252 = Bundle(cluster=w395, "Color"=w408) -> (w403:T4)  [unwired: 1 in]
                n253 = Bundle(cluster=w395, "Color"=w407) -> (w404:T4)  [unwired: 1 in]
                n254 = Bundle(cluster=w395, "Color"=w406) -> (w405:T4)  [unwired: 1 in]
                n255 = local write "_TunnelsAndTerminalsColors"(w405) -> ()
                n256 = To Unsigned Word Integer(number=w397) -> (unsigned 16bit integer=w396:u16)
                n257 = To Unsigned Word Integer(number=w399) -> (unsigned 16bit integer=w398:u16)
                n258 = local write "_CenterThickness"(w398) -> ()
                n259 = local write "_EdgeThickness"(w396) -> ()
                n260 = local write "_CenterPattern"(w401) -> ()
                n261 = local write "_CenterColor1"(w403) -> ()
                n262 = local write "_CenterColor2"(w404) -> ()
                n263 = local write "_EdgeColor"(w402) -> ()
              }
              frame -1 {
              }
            }
          }
          event "DeleteWireStyle": Value Change {
            n264 = event-data() -> ()  [unwired: 1 in, 6 out]
            n265 = local read "WireStyleList"() -> (w415:T2[])
            n266 = for {
              tunnel: w415 -> [w422] mode=indexing
              tunnel: [w420] -> w414
              tunnel: [w419] -> _
              tunnel: [w418] -> w413
              i -> [w419]
              stop <- w418 stop-if-true
              n267 = Unbundle By Name(w422) -> ("Name"=w420:string, "Status"=w421:u16)
              n268 = Not Equal To 0?(x=w421) -> (x != 0?=w418:bool)
            }
            n269 = case shown="True" w413 {
              tunnel: w414 -> [_ w416]
              frame False {
              }
              frame True {
                n270 = call "BaseProvider_WireStylesManager.vi"("Action(Read)"=enum16{"Read", "UpdateOne", "DeleteOne"}."DeleteOne", "WireStyleName(Default)"=w416) -> ()  [unwired: 6 in, 4 out]
              }
            }
          }
          event "Update/AddWireStyle": Value Change {
            n271 = event-data() -> ()  [unwired: 1 in, 6 out]
            n272 = Unbundle By Name(w427) -> ("CurrentWireStyle"=w426:T8)
            n273 = local read "WireStyleName"() -> (w424:string)
            n274 = call "BaseProvider_WireStylesManager.vi"("Action(Read)"=enum16{"Read", "UpdateOne", "DeleteOne"}."UpdateOne", "WireConfiguration(New or Updating)"=w426, "WireStyleName(Default)"=w424) -> ()  [unwired: 5 in, 4 out]
          }
          event "Up", "Down": Value Change {
            n275 = event-data() -> ()  [unwired: 1 in, 6 out]
            n276 = local read "WireStyleList"() -> (w438:T2[])
            n277 = Unbundle By Name(w441) -> ("CurrentWireStyle"=w440:T8)
            n278 = for {
              tunnel: w438 -> [w446] mode=indexing
              tunnel: [w443] -> w429
              tunnel: [w442] -> w436
              i -> [w442]
              stop <- w444 stop-if-true
              n279 = Unbundle By Name(w446) -> ("Name"=w443:string, "Status"=w445:u16)
              n280 = Not Equal To 0?(x=w445) -> (x != 0?=w444:bool)
            }
            n281 = Increment(x=w436) -> (x+1=w437:i32)
            n282 = Decrement(x=w436) -> (x-1=w435:i32)
            n283 = Select(t=w437, s="Down", f=w435) -> (s? t:f=w431:i32)
            n284 = call "BaseProvider_WireStylesManager.vi"("Action(Read)"=enum16{"Read", "UpdateOne", "DeleteOne"}."UpdateOne", "NewIndex(-1=NoChange/Inserted Last If not found)"=w431, "WireConfiguration(New or Updating)"=w440, "WireStyleName(Default)"=w429) -> ("AllWireConfigurations(Names)"=w430:string[])  [unwired: 4 in, 3 out]
            n285 = Search 1D Array(1D array=w430, element=w429) -> (index of element=w428:i32)  [unwired: 1 in]
            n286 = Format Into String(format string="UpdateWirePreView\nUpdateWireStyleList>>%d\nUpdate", w428) -> (resulting string=w432:string)  [unwired: 2 in, 1 out]
          }
          event "_Dice": Mouse Enter {
            n287 = event-data() -> ()  [unwired: 1 in, 1 out]
            n288 = local write "_Dice"(cluster{"Boolean 2":bool, "Dice":bool} {"Boolean 2"=TRUE, "Dice"=FALSE} ("Dice")) -> ()
          }
          event "_Dice": Mouse Leave {
            n289 = event-data() -> ()  [unwired: 1 in, 1 out]
            n290 = local write "_Dice"(cluster{"Boolean 2":bool, "Dice":bool} {"Boolean 2"=FALSE, "Dice"=FALSE} ("Dice")) -> ()
          }
          event "_HelpDefaultConfiguration": Value Change {
            n291 = event-data() -> ()  [unwired: 1 in, 1 out]
            n292 = fn#1354() -> (1:w452:bool)  [unwired: 1 out]
            n293 = Not(x=w452) -> (.not. x?=w451:bool)
            n294 = Control Help Window(1:w451) -> ()  [unwired: 1 in]
          }
        }
      }
      frame "UpdateClass" {
        n295 = local read "_CenterColor1"() -> (w475:T4)
        n296 = local read "_CenterColor2"() -> (w479:T4)
        n297 = local read "_EdgeColor"() -> (w477:T4)
        n298 = local read "_EdgeThickness"() -> (w481:T7)
        n299 = local read "_CenterThickness"() -> (w476:T6)
        n300 = local read "_TunnelsAndTerminalsColors"() -> (w474:T4)
        n301 = local read "_CenterPattern"() -> (w484:T5)
        n302 = Format Into String("_DefaultConnectorPanePattern") -> (resulting string=w457:string)  [unwired: 3 in, 1 out]
        n303 = Unbundle By Name(w489) -> ("ClassRefCreated"=w491:bool, "ClassRef"=w456:refnum<vi>)
        n304 = disable-structure shown="Enabled" {
          disable-tunnel: [w500 _] -> w469
          frame Enabled {
            n305 = property on="_Icon" class="Ring (strict)"() -> ("Strings []"=w502:string[])  [unwired: 2 in, 2 out]
            n306 = local read "_Icon"() -> (w501:u16)
            n307 = Index Array(array=w502, index=w501) -> (element=w500:string)
          }
          frame Disabled {
          }
        }
        n308 = To Unsigned Long Integer(number=w476) -> (unsigned 32bit integer=w478:u32)
        n309 = Unbundle(w475) -> ("Color"=w485:u32)  [unwired: 1 out]
        n310 = Unbundle(w479) -> ("Color"=w486:u32)  [unwired: 1 out]
        n311 = Unbundle(w474) -> ("Color"=w487:u32)  [unwired: 1 out]
        n312 = Unbundle(w477) -> ("Color"=w482:u32)  [unwired: 1 out]
        n313 = Increment(x=w478) -> (x+1=w483:u32)
        n314 = call "GDSLvClass_ReadClassType.vi"("Class Refnum In"=w456, "error in (no error)"=w461) -> ("Class Refnum Out"=w463:refnum<vi>, "ClassSettings"=w460:T14, "error out"=w464:errorcluster)  [unwired: 15 in]
        n315 = Bundle By Name(cluster=w460, "ConnectorPanePattern"=w457) -> (w459:T14)
        n316 = call "GDSLvClass_StoreClassType.vi"("Class Refnum In"=w463, "ClassSettings"=w459, "error in (no error)"=w464) -> ("Class Refnum Out"=w455:refnum<vi>, "error out"=w462:errorcluster)  [unwired: 15 in]
        n317 = Bundle(cluster=T8 {"Edge thickness"=0, "Edge color"=0, "Center thickness"=0, "Center pattern"=enum."Solid", "CenterColor1"=0, "CenterColor2"=0, "Tunnels and terminals colors"=0} ("WireConfiguration"), "Edge thickness"=w481, "Edge color"=w482, "Center thickness"=w483, "Center pattern"=w484, "CenterColor1"=w485, "CenterColor2"=w486, "Tunnels and terminals colors"=w487) -> (w473:T8)
        n318 = disable-structure shown="Enabled" {
          disable-tunnel: w469 -> [w498 _]
          disable-tunnel: [w495 w499] -> w454
          disable-tunnel: w462 -> [w497 w499]
          disable-tunnel: w455 -> [w496 _]
          frame Enabled {
            n319 = call "GDSLvClass_StoreClassItemIcon.vi"("Library Refnum"=w496, "ClassItemIconName"=w498, "error in (no error)"=w497) -> ("error out"=w495:errorcluster)  [unwired: 15 in, 1 out]
          }
          frame Disabled {
          }
        }
        n320 = call "GOOP_WirePenTranslator.vi"("WireConfigurationIn"=w473) -> ("WirePensOut"=w488:T17)  [unwired: 17 in, 1 out]
        n321 = property class="LVClassLibrary"(reference=w455, error in=w454, "Wire Pens"=w488) -> (reference out=w472:refnum<vi>, error out=w471:errorcluster)
        n322 = invoke class="LVClassLibrary" method="Save"(reference=w472, error in=w471) -> (reference out=w470:refnum<vi>, error out=w466:errorcluster)  [unwired: 2 in, 2 out]
        n323 = case shown="True" w491 {
          tunnel: w466 -> [w506 w509]
          tunnel: w470 -> [_ w508]
          tunnel: [w506 w507] -> w465
          frame False {
          }
          frame True {
            n324 = Close Reference(reference=w508, error in (no error)=w509) -> (error out=w507:errorcluster)
          }
        }
        n325 = Unbundle By Name(w465) -> ("code"=w468:i32)
        n326 = case shown="Default" w468 {
          tunnel: w461 -> [w503 _]
          tunnel: [w503 w505] -> w467
          tunnel: w465 -> [_ w505]
          frame 8 {
            n327 = One Button Dialog(message="Warning\nThe changes could not be saved.\nThe file might be read-only.") -> ()  [unwired: 1 in, 1 out]
          }
          frame Default {
          }
        }
        n328 = Select(t="SaveConfiguration", s="_SetToDefaultForAllClasses", f="Exit") -> (s? t:f=w494:string)
      }
      frame "UpdateIconPreview" {
        n329 = property on="_Icon" class="Ring (strict)"() -> ("Strings []"=w513:string[])  [unwired: 2 in, 2 out]
        n330 = local read "_Icon"() -> (w512:u16)
        n331 = Index Array(array=w513, index=w512) -> (element=w511:string)
        n332 = call "GOOP_GetOverlayIconPath.vi"("IconName(NoPngExtension)"=w511) -> ("IconPath"=w510:path)  [unwired: 10 in]
        n333 = Empty String/Path?(string/path=w510) -> (empty?=w514:bool)
        n334 = case shown="False" w514 {
          tunnel: w510 -> [w518 _]
          frame False {
            n335 = call <vilib>:"Read PNG File.vi"("path to PNG file"=w518) -> ("image data"=w521:T19)  [unwired: 8 in, 2 out]
            n336 = call "GOOP_DrawWirePreview_ZoomImage.vi"("image data 2"=w521, "Zoom"=5) -> ("image data"=w522:T19)
            n337 = call <vilib>:"Draw Flattened Pixmap.vi"("image data"=w522) -> ("new picture"=→"_Preview":picture)  [unwired: 8 in]
          }
          frame True {
          }
        }
      }
      frame "SaveConfiguration" {
        n338 = local read "_CenterColor1"() -> (w539:T4)
        n339 = local read "_CenterColor2"() -> (w538:T4)
        n340 = local read "_EdgeColor"() -> (w542:T4)
        n341 = local read "_EdgeThickness"() -> (w543:T7)
        n342 = local read "_CenterThickness"() -> (w541:T6)
        n343 = local read "_TunnelsAndTerminalsColors"() -> (w537:T4)
        n344 = local read "_CenterPattern"() -> (w540:T5)
        n345 = local read "_DefaultConnectorPanePattern"() -> (w532:T3)
        n346 = property on="_Icon" class="Ring (strict)"() -> ("Strings []"=w529:string[])  [unwired: 2 in, 2 out]
        n347 = local read "_Icon"() -> (w530:u16)
        n348 = Index Array(array=w529, index=w530) -> (element=w528:string)
        n349 = To Unsigned Long Integer(number=w541) -> (unsigned 32bit integer=w550:u32)
        n350 = case shown="True" w531 {
          tunnel: [w551 w557] -> w527
          tunnel: w528 -> [w551 w552]
          frame False {
          }
          frame True {
            n351 = call "BaseProvider_IniFileSettings.vi"() -> ("IniFileSettings"=w555:T13, "error out"=w553:errorcluster)  [unwired: 18 in]
            n352 = Bundle By Name(cluster=w555, "InterfaceIcon"=w552) -> (w556:T13)
            n353 = call "BaseProvider_ConfigurationMemory.vi"() -> ("IconOut"=w557:string)  [unwired: 13 in, 6 out]
            n354 = call "BaseProvider_IniFileSettings.vi"("IniFileSettings"=w556, "error in (no error)"=w553, "Action"=enum16{"Read", "Load", "Save"}."Save") -> ()  [unwired: 15 in, 2 out]
          }
        }
        n355 = Increment(x=w550) -> (x+1=w549:u32)
        n356 = Unbundle(w539) -> ("Color"=w547:u32)  [unwired: 1 out]
        n357 = Unbundle(w538) -> ("Color"=w548:u32)  [unwired: 1 out]
        n358 = Unbundle(w537) -> ("Color"=w545:u32)  [unwired: 1 out]
        n359 = Unbundle(w542) -> ("Color"=w546:u32)  [unwired: 1 out]
        n360 = Bundle By Name(cluster=T8 {"Edge thickness"=0, "Edge color"=0, "Center thickness"=0, "Center pattern"=enum."Solid", "CenterColor1"=0, "CenterColor2"=0, "Tunnels and terminals colors"=0} ("WireConfiguration"), "Edge thickness"=w543, "Edge color"=w546, "Center thickness"=w549, "Center pattern"=w540, "CenterColor1"=w547, "CenterColor2"=w548, "Tunnels and terminals colors"=w545) -> (w525:T8)
        n361 = call "BaseProvider_WireStylesManager.vi"() -> ("AllWireConfigurations"=w526:T8[])  [unwired: 8 in, 3 out]
        n362 = call "BaseProvider_ConfigurationMemory.vi"("WireConfiguration"=w525, "Icon"=w527, "Action"=enum16{"Read", "Load", "Save"}."Save", "PatternIn"=w532) -> ()  [unwired: 9 in, 7 out]
        n363 = Search 1D Array(1D array=w526, element=w525) -> (index of element=w523:i32)  [unwired: 1 in]
        n364 = Bundle By Name(cluster=w534, "SelectedWireStyleIndex"=w523) -> (w524:T9)
      }
    }
  }
  "Error Out" <- w34
  n365 = Generate User Event(user event=w32, event data cluster="Stop" ("Stop")) -> (user event out=w33:refnum<user-event>)  [unwired: 2 in, 1 out]
  n366 = Destroy User Event(user event=w33) -> (error out=w21:errorcluster)  [unwired: 1 in]
  n367 = Destroy User Event(user event=w19, error in=w21) -> (error out=w20:errorcluster)
  n368 = case shown="False" "OnlyWireStyleConfiguration(False)" {
    tunnel: w27 -> [w564 _]
    tunnel: w24 -> [w562 _]
    tunnel: w19 -> [w561 _]
    tunnel: w18 -> [w560 _]
    tunnel: w17 -> [w559 _]
    frame False {
      n369 = case shown="False" w560 {
        tunnel: [CommonVIs_ClassIconSelection_Action."All" ("IconsToShow(All)") CommonVIs_ClassIconSelection_Action."Only Interface" ("IconsToShow(All)")] -> w566
        frame False {
        }
        frame True {
        }
      }
      n370 = control-ref of="IconSelection"() -> (w563:refnum<vi>)
      n371 = control-ref of="Icon"() -> (w565:refnum<vi>)
      n372 = call "CommonVIs_ClassIconSelection.vi"("SaveChangesInClassRightAway(True)"=FALSE, "IconSelected"=w561, "IconsToShow(All)"=w566, "Icon"=w565, "error in (no error)"=w559, "Messages(Stop or Empty string will stop this VI)"=w564, "IconSelection"=w563, "LVClassToActOn"=w562) -> ()  [unwired: 4 in]
    }
    frame True {
    }
  }
  n373 = Unregister For Events(event registration refnum=w22, error in=w20) -> ()  [unwired: 1 out]
  n374 = call "GDSString_AddStatesToQueue.vi"() -> ()  [unwired: 15 in, 1 out]
  n375 = Unbundle By Name(w3) -> ("SelectedWireStyleIndex"=→"SelectedWireStyleIndex":i32)
